vi "CreateEventOnError.vi"(8 "error in (no error)":errorcluster, 11 "User Event in":refnum<user-event>) -> (0 "error out":errorcluster)   [LabVIEW 2020]
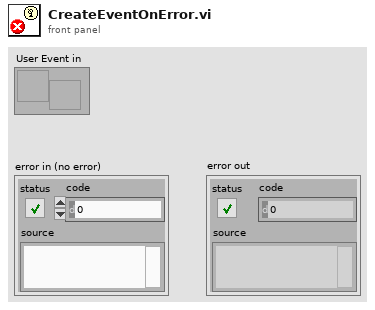
[diagram p1: front panel]
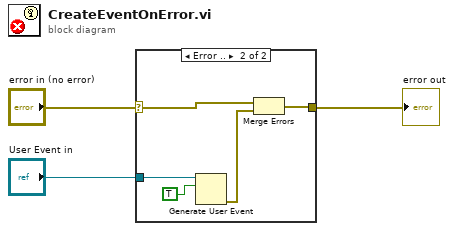
[diagram p0: block diagram]
diagram:
  n1 = case shown="Error .." "error in (no error)" {
    selector: "error in (no error)" -> [w4 w7]
    tunnel: [w4 w9] -> w1
    tunnel: "User Event in" -> [_ w5]
    frame No Error {
    }
    frame Error {
      n2 = Generate User Event(user event=w5, event data cluster=TRUE ("event data")) -> (error out=w8:errorcluster)  [unwired: 2 in, 1 out]
      n3 = Merge Errors(w7, w8) -> (w9:errorcluster)
    }
  }
  "error out" <- w1
